vi "aal_Complex Modulator with Phase (real input).vi"(7 "reset ?":bool, 8 "initial phase":dbl, 9 "fs":dbl=1024.0 min=-0.5 max=0.5 format="%.2f", 10 "frequency":dbl min=-0.5 max=0.5 format="%.2f", 11 "x":dbl[](array[numeric])) -> (3 "y":cdb[](array[numeric]))   [LabVIEW 2020, in "NI_AAL_SigProc.lvlib"]
doc: "Modulates the signal to frequency. The center frequency should be normalized (-0.5, 0.5)."
uses:
  <vilib>/Analysis/NI_AAL_SigProc.lvlib
  <resource>/lvanlys.dll
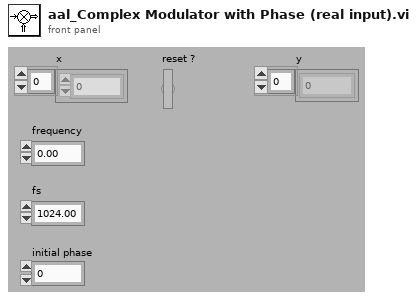
[diagram p1: front panel]
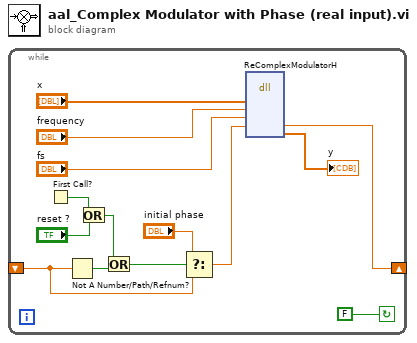
[diagram p0: block diagram]
diagram:
  n1 = while {
    shift-left: _ -> [w13]
    shift-right: [w8] -> _
    stop <- FALSE continue-if-true
    n2 = First Call?() -> (First Call?: T/F=w4:bool)
    n3 = Not A Number/Path/Refnum?(number/path/refnum=w13) -> (NaN/Path/Refnum?=w14:bool)
    n4 = Or(x=w4, y="reset ?") -> (x .or. y?=w2:bool)
    n5 = Or(x=w2, y=w14) -> (x .or. y?=w7:bool)
    n6 = Select(t="initial phase", s=w7, f=w13) -> (s? t:f=w9:dbl)
    n7 = dll-call lib="e:/builds/penguin/labview/branches/2020/dev/dist/resource/lvanlys.*" fn="ReComplexModulatorH"("x"="x", "fc"="frequency", "fs"="fs", "initial_phase"=w9) -> ("initial_phase"=w8:dbl, "y"=→"y":cdb[])  [unwired: 8 in, 2 out]
  }
